vi "擦除盲元表.vi"(8 "error in":errorcluster, 10 "分辨率":string, 11 "address":u32) -> (0 "error out":errorcluster, 2 "return":i32)   [LabVIEW 2016]
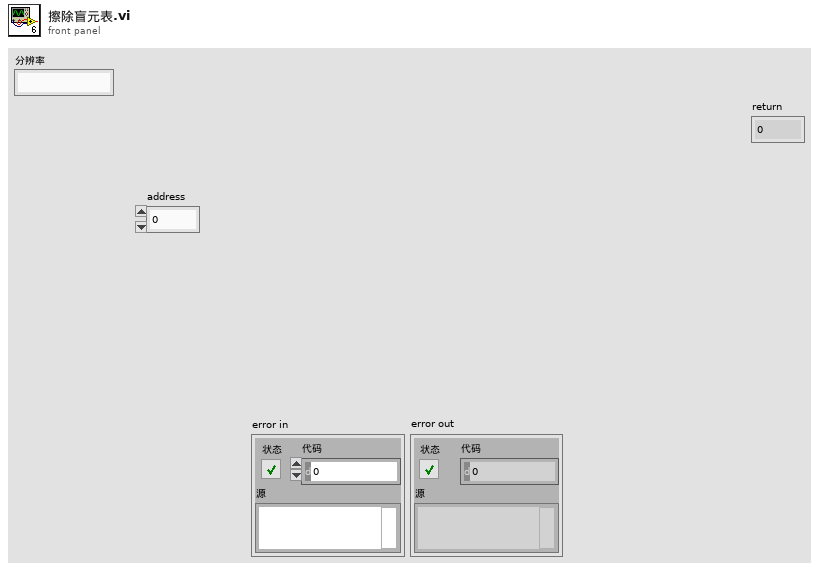
[diagram p1: front panel]
types:
  T1 = cluster{"byCmdType":u8, "bySubCmd":u8, "byPara":u8, "byAddr_h":u8, "byAddr_l":u8, "byAddr_ll":u8, "byLen_h":u8, "byLen_l":u8}
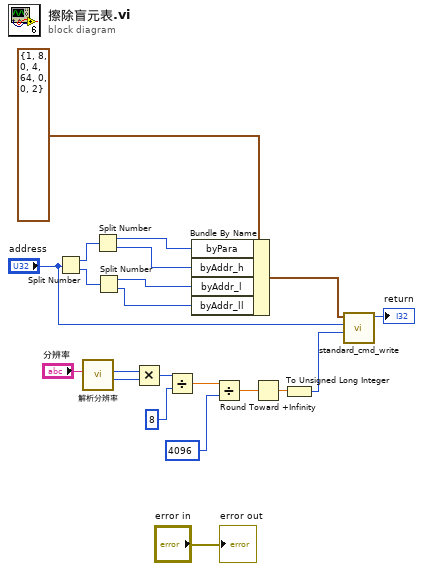
[diagram p0: block diagram]
diagram:
  n1 = Split Number(x="address") -> (hi(x)=w8:u16, lo(x)=w7:u16)
  n2 = call "解析分辨率.vi"("分辨率"="分辨率") -> ("number 2"=w17:i32, "number"=w18:i32)  [unwired: 9 in]
  n3 = Split Number(x=w8) -> (hi(x)=w6:u8, lo(x)=w5:u8)
  n4 = Split Number(x=w7) -> (hi(x)=w4:u8, lo(x)=w3:u8)
  n5 = Multiply(x=w18, y=w17) -> (x*y=w16:i32)
  n6 = Divide(x=w16, y=8) -> (x/y=w14:dbl)
  n7 = Bundle By Name(cluster=T1 {"byCmdType"=1, "bySubCmd"=8, "byPara"=0, "byAddr_h"=4, "byAddr_l"=64, "byAddr_ll"=0, "byLen_h"=0, "byLen_l"=2} ("cmd_std_header_t"), "byPara"=w6, "byAddr_h"=w5, "byAddr_l"=w4, "byAddr_ll"=w3) -> (w2:T1)
  n8 = Divide(x=w14, y=4096) -> (x/y=w12:dbl)
  n9 = Round Toward +Infinity(x=w12) -> (ceil(x): smallest int >= x=w11:dbl)
  n10 = To Unsigned Long Integer(number=w11) -> (unsigned 32bit integer=w10:u32)
  n11 = call "standard_cmd_write.vi"("dwLen"=w10, "dwAddr"="address", "cmd_std_header_t"=w2) -> ("return"=→"return":i32)  [unwired: 7 in, 1 out]
  "error out" <- "error in"
